vi "v4.vi"() -> ()   [LabVIEW 2015]
uses:
  <vilib>/Analysis/3filter.llb/Filter Passband Type.ctl
  <vilib>/Instr/_visa.llb/VISA Configure Serial Port (Instr).vi
  <vilib>/Analysis/3filter.llb/Butterworth Filter (DBL).vi
  <vilib>/Analysis/NI_AALBase.lvlib
panel:
  in  "Tab Control":enum32{"Configurações", "Gráficos"}(tab)
  in  "stop":bool
  in  "PORTA COM":refnum<visa-resource-name>
  in  "Digite aqui o endereço e nome do arquivo":string
  out "Max_Direito":dbl format="%#_3g"
  out "Max_esquerdo":dbl format="%#_3g"
  out "Angulo_E":dbl format="%#_3g"
  out "Tempo_D":dbl format="%#_3g"
  out "Angulo_D":dbl format="%#_3g"
  out "Tempo_E":dbl format="%#_3g"
  in  "milliseconds to wait":u32=1000
  out "Left":cluster{"X":dbl[], "Y":dbl[]}[](graph)
  out "Right":cluster{"X":dbl[], "Y":dbl[]}[](graph)
  out "angle 2":cluster{"X":dbl[], "Y":dbl[]}[](graph)
  out "angle_fil":dbl[](array[numeric])
  out "right_fil":dbl[](array[numeric])
  out "angle":dbl[](array[numeric])
  out "right":dbl[](array[numeric])
  out "left_Fil":dbl[](array[numeric])
  out "left":dbl[](array[numeric])
  out "Tempo":dbl[](array[numeric])
  out "Array_left":dbl[](array[numeric])
  out "Array_right":dbl[](array[numeric])
  out "Array_angle":dbl[](array[numeric])
  out "Tempo1":dbl[](array[numeric])
  # "Tempo para começar (ms)"
  # "Direito"
  # "Esquerdo"
  # "FORÇA MÁX."
  # "ÂNGULO"
  # "TEMPO"
  # "Desenvolvido por Tércio Apolinário-Souza"
  # "Esquerdo"
  # "Direito"
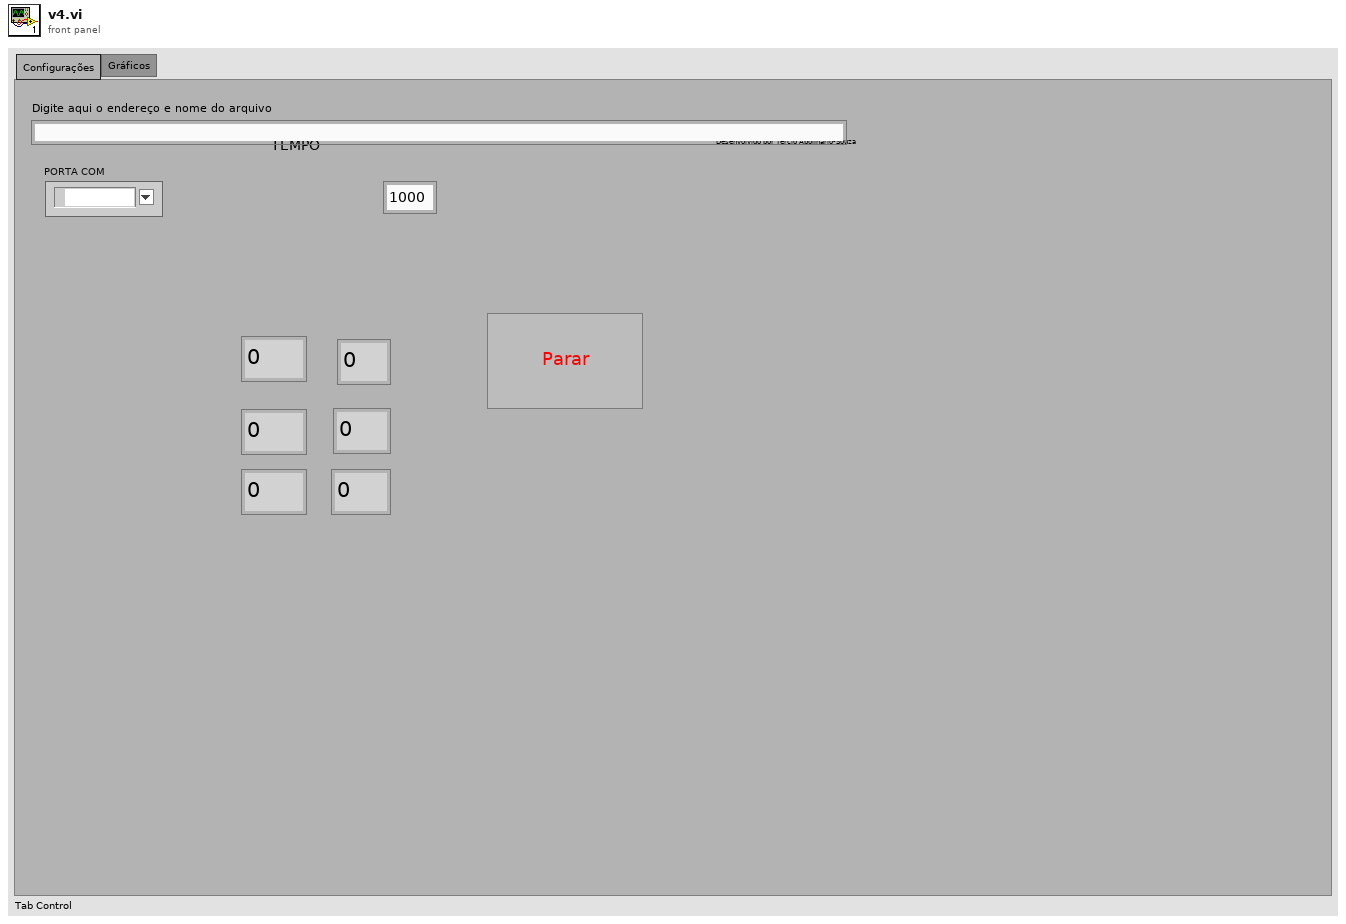
[diagram p1: front panel]
types:
  T1 = typedef "NI_AALBase.lvlib/Filter Passband Type.ctl" = enum32{"Lowpass", "Highpass", "Bandpass", "Bandstop"}
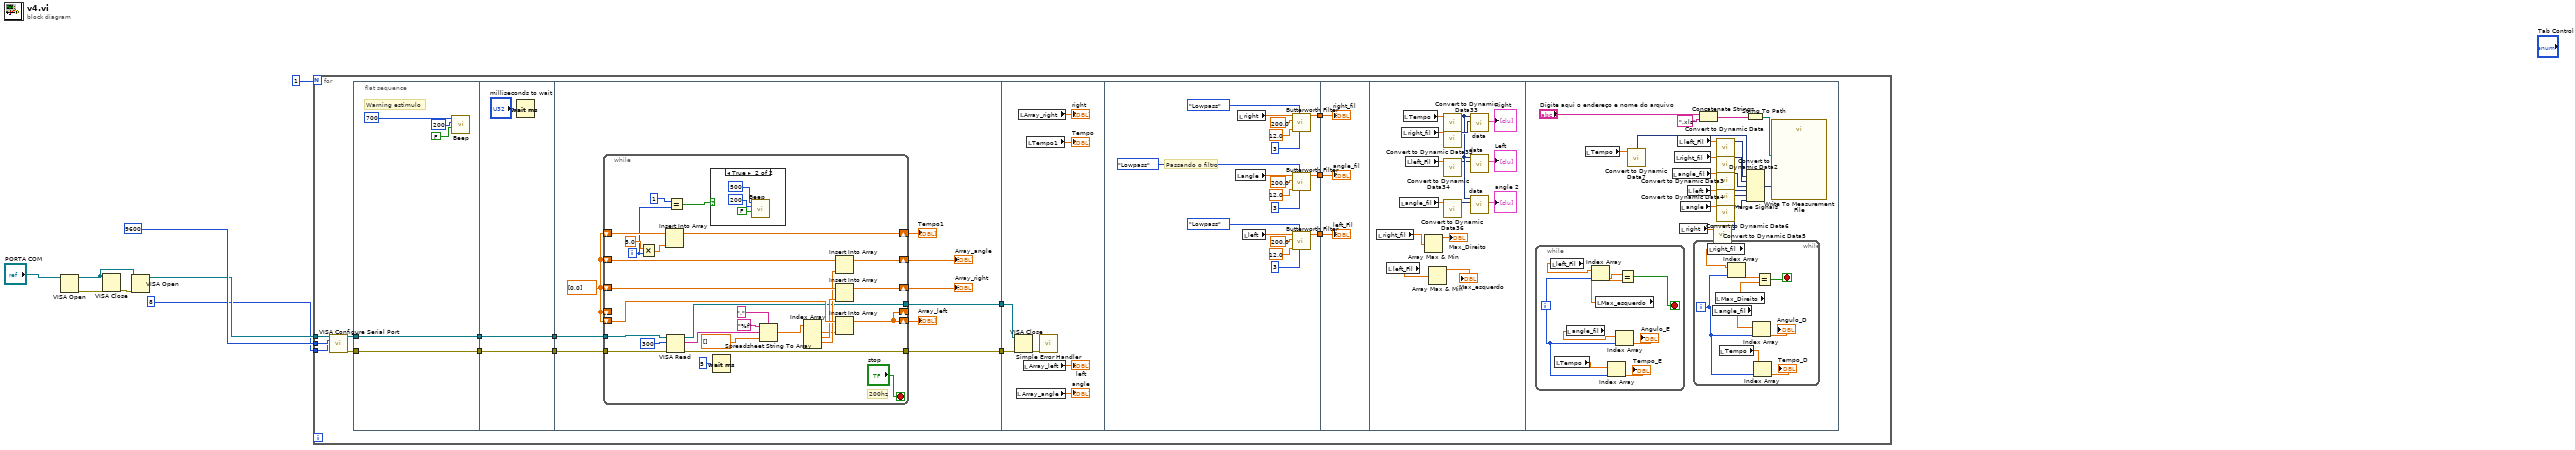
[diagram p0: block diagram]
diagram:
  n1 = VISA Open(VISA resource name="PORTA COM") -> (VISA resource name=w6:refnum<visa-resource-name>, error out=w5:errorcluster)  [unwired: 4 in]
  n2 = VISA Close(VISA resource name=w6, error in (no error)=w5) -> (error out=w4:errorcluster)
  n3 = VISA Open(error in (no error)=w4, VISA resource name=w6) -> (VISA resource name=w3:refnum<visa-resource-name>)  [unwired: 3 in, 1 out]
  n4 = for {
    N: 1 -> [_]
    tunnel: u32 9600 ("baud rate (9600)") -> [w22]
    tunnel: w3 -> [w21]
    tunnel: u16 8 ("data bits (8)") -> [w20]
    n5 = call-poly "VISA Configure Serial Port"("VISA resource name"=w21, "baud rate (9600)"=w22, "data bits (8)"=w20) -> ("VISA resource name out"=w19:refnum<visa-resource-name>, "error out"=w18:errorcluster)  [unwired: 11 in]
    n6 = flat-sequence {
      tunnel: [w23] -> w12
      tunnel: [w24] -> w11
      tunnel: w19 -> [w24]
      tunnel: w18 -> [w23]
      tunnel: w12 -> [w30]
      tunnel: [w30] -> w10
      tunnel: w11 -> [w29]
      tunnel: [w29] -> w9
      tunnel: w9 -> [w39]
      tunnel: [w37] -> w17
      tunnel: w10 -> [w38]
      tunnel: [w36] -> w16
      tunnel: w17 -> [w76]
      tunnel: w16 -> [w75]
      tunnel: [w80] -> w15
      tunnel: [w79] -> w14
      tunnel: [w78] -> w13
      tunnel: w15 -> [w98]
      tunnel: w14 -> [w97]
      tunnel: w13 -> [w96]
      frame #0 {
        # "Warning estimulo"
        n7 = call <vilib>:"Beep.vi"("use system alert? (T)"=FALSE, "duration (msec)"=u32 200, "frequency (Hz)"=u32 700) -> ()  [unwired: 9 in]
      }
      frame #1 {
        n8 = Wait (ms)(milliseconds to wait="milliseconds to wait") -> ()  [unwired: 1 out]
      }
      frame #2 {
        w32 = dbl[] [0.0] ("appended array")
        n9 = while {
          tunnel: w39 -> [w64]
          tunnel: w38 -> [w63]
          tunnel: [w50] -> w37
          tunnel: [w62] -> w36
          shift-right: [w46] -> w33
          shift-left: w32 -> [w59]
          shift-right: [w51] -> w34
          shift-left: w32 -> [w57]
          shift-right: [w49] -> w35
          shift-left: w32 -> [w56]
          shift-right: [w52] -> w31
          shift-left: w32 -> [w48]
          shift-right: [w46] -> _
          shift-left: w32 -> [_]
          i -> [w42]
          stop <- "stop" stop-if-true
          # "200hz"
          n10 = Multiply(x=5.0, y=w42) -> (x*y=w45:dbl)
          n11 = Insert Into Array(array=w48, new element=w45) -> (w52:dbl[])  [unwired: 1 in]
          n12 = VISA Read(VISA resource name=w64, byte count=u32 300, error in (no error)=w63) -> (VISA resource name out=w50:refnum<visa-resource-name>, read buffer=w60:string, error out=w62:errorcluster)  [unwired: 1 out]
          n13 = Equal?(x=1, y=w42) -> (x = y?=w40:bool)
          n14 = case shown="True" w40 {
            frame False {
            }
            frame True {
              n15 = call <vilib>:"Beep.vi"("use system alert? (T)"=FALSE, "duration (msec)"=u32 200, "frequency (Hz)"=u32 500) -> ()  [unwired: 9 in]
            }
          }
          n16 = Wait (ms)(milliseconds to wait=u32 5 ("millisecond multiple")) -> ()  [unwired: 1 out]
          n17 = Spreadsheet String To Array(delimiter (Tab)=",", format string="%f", spreadsheet string=w60, array type (2D Dbl)=dbl[] []) -> (array=w54:dbl[])
          n18 = Index Array(array=w54) -> (element #1=w53:dbl, element #2=w58:dbl, element #3=w55:dbl)  [unwired: 4 in, 1 out]
          n19 = Insert Into Array(array=w56, new element=w55) -> (w49:dbl[])  [unwired: 1 in]
          n20 = Insert Into Array(array=w57, new element=w58) -> (w51:dbl[])  [unwired: 1 in]
          n21 = Insert Into Array(array=w59, new element=w53) -> (w46:dbl[])  [unwired: 1 in]
        }
        "Tempo1" <- w31
        "Array_angle" <- w35
        "Array_right" <- w34
        "Array_left" <- w33
      }
      frame #3 {
        n22 = VISA Close(VISA resource name=w76, error in (no error)=w75) -> (error out=w77:errorcluster)
        n23 = local read "Array_angle"() -> (→"angle":dbl[])
        n24 = local read "Array_right"() -> (→"right":dbl[])
        n25 = local read "Array_left"() -> (→"left":dbl[])
        n26 = local read "Tempo1"() -> (→"Tempo":dbl[])
        n27 = call <vilib>:"Simple Error Handler.vi"("error in (no error)"=w77) -> ()  [unwired: 1 in, 8 out]
      }
      frame #4 {
        # "Passando o filtro"
        n28 = local read "angle"() -> (w81:dbl[])
        n29 = local read "right"() -> (w82:dbl[])
        n30 = local read "left"() -> (w91:dbl[])
        n31 = call-poly <vilib>:"Butterworth Filter.vi"("order"=3, "filter type"=Filter_Passband_Type."Lowpass", "low cutoff freq: fl"=12.0, "sampling freq: fs"=200.0, "X"=w82) -> ("Filtered X"=w79:dbl[])  [unwired: 3 in, 1 out]
        n32 = call-poly <vilib>:"Butterworth Filter.vi"("order"=3, "filter type"=Filter_Passband_Type."Lowpass", "low cutoff freq: fl"=12.0, "sampling freq: fs"=200.0, "X"=w81) -> ("Filtered X"=w78:dbl[])  [unwired: 3 in, 1 out]
        n33 = call-poly <vilib>:"Butterworth Filter.vi"("order"=3, "filter type"=Filter_Passband_Type."Lowpass", "low cutoff freq: fl"=12.0, "sampling freq: fs"=200.0, "X"=w91) -> ("Filtered X"=w80:dbl[])  [unwired: 3 in, 1 out]
      }
      frame #5 {
        "left_Fil" <- w98
        "right_fil" <- w97
        "angle_fil" <- w96
      }
      frame #6 {
        n34 = local read "right_fil"() -> (w102:dbl[])
        n35 = local read "left_Fil"() -> (w100:dbl[])
        n36 = local read "angle_fil"() -> (w103:dbl[])
        n37 = local read "right_fil"() -> (w104:dbl[])
        n38 = local read "Tempo"() -> (w106:dbl[])
        n39 = local read "left_Fil"() -> (w105:dbl[])
        n40 = Array Max & Min(array=w102) -> (max value=→"Max_Direito":dbl)  [unwired: 3 out]
        n41 = Array Max & Min(array=w100) -> (max value=→"Max_esquerdo":dbl)  [unwired: 3 out]
        n42 = call "Convert to Dynamic Data33"("Array"=w106) -> ("Dynamic Data Type"=w111:dynamicdata)  [unwired: 3 in]
        n43 = call "Convert to Dynamic Data35"("Array"=w104) -> ("Dynamic Data Type"=w113:dynamicdata)  [unwired: 3 in]
        n44 = call "Convert to Dynamic Data34"("Array"=w105) -> ("Dynamic Data Type"=w107:dynamicdata)  [unwired: 3 in]
        n45 = call "Convert to Dynamic Data36"("Array"=w103) -> ("Dynamic Data Type"=w112:dynamicdata)  [unwired: 3 in]
        n46 = call "data"("Y Input"=w113, "X Input"=w111) -> ("XY Graph"=→"Right":cluster{"X":dbl[], "Y":dbl[]}[])  [unwired: 8 in, 1 out]
        n47 = call "data"("Y Input"=w107, "X Input"=w111) -> ("XY Graph"=→"Left":cluster{"X":dbl[], "Y":dbl[]}[])  [unwired: 8 in, 1 out]
        n48 = call "data"("Y Input"=w112, "X Input"=w111) -> ("XY Graph"=→"angle 2":cluster{"X":dbl[], "Y":dbl[]}[])  [unwired: 8 in, 1 out]
      }
      frame #7 {
        n49 = while {
          i -> [w143]
          stop <- w147 stop-if-true
          n50 = local read "left_Fil"() -> (w150:dbl[])
          n51 = local read "Tempo"() -> (w144:dbl[])
          n52 = local read "angle_fil"() -> (w146:dbl[])
          n53 = Index Array(array=w150, index=w143) -> (element=w149:dbl)
          n54 = local read "Max_esquerdo"() -> (w148:dbl)
          n55 = Index Array(array=w144, index=w143) -> (element=→"Tempo_E":dbl)
          n56 = Index Array(array=w146, index=w143) -> (element=→"Angulo_E":dbl)
          n57 = Equal?(x=w149, y=w148) -> (x = y?=w147:bool)
        }
        n58 = local read "Tempo"() -> (w115:dbl[])
        n59 = call "Convert to Dynamic Data7"("Array"=w115) -> ("Dynamic Data Type"=w114:dynamicdata)  [unwired: 3 in]
        n60 = local read "angle_fil"() -> (w123:dbl[])
        n61 = local read "right_fil"() -> (w125:dbl[])
        n62 = local read "left_Fil"() -> (w127:dbl[])
        n63 = local read "right"() -> (w119:dbl[])
        n64 = local read "angle"() -> (w117:dbl[])
        n65 = local read "left"() -> (w121:dbl[])
        n66 = while {
          i -> [w134]
          stop <- w138 stop-if-true
          n67 = local read "right_fil"() -> (w141:dbl[])
          n68 = local read "angle_fil"() -> (w137:dbl[])
          n69 = local read "Max_Direito"() -> (w139:dbl)
          n70 = local read "Tempo"() -> (w135:dbl[])
          n71 = Index Array(array=w141, index=w134) -> (element=w140:dbl)
          n72 = Index Array(array=w137, index=w134) -> (element=→"Angulo_D":dbl)
          n73 = Index Array(array=w135, index=w134) -> (element=→"Tempo_D":dbl)
          n74 = Equal?(x=w140, y=w139) -> (x = y?=w138:bool)
        }
        n75 = Concatenate Strings("Digite aqui o endereço e nome do arquivo", ".xls" ("string")) -> (w129:string)
        n76 = call "Convert to Dynamic Data5"("Array"=w119) -> ("Dynamic Data Type"=w118:dynamicdata)  [unwired: 3 in]
        n77 = call "Convert to Dynamic Data"("Array"=w127) -> ("Dynamic Data Type"=w126:dynamicdata)  [unwired: 3 in]
        n78 = call "Convert to Dynamic Data2"("Array"=w125) -> ("Dynamic Data Type"=w124:dynamicdata)  [unwired: 3 in]
        n79 = call "Convert to Dynamic Data3"("Array"=w123) -> ("Dynamic Data Type"=w122:dynamicdata)  [unwired: 3 in]
        n80 = call "Convert to Dynamic Data4"("Array"=w121) -> ("Dynamic Data Type"=w120:dynamicdata)  [unwired: 3 in]
        n81 = call "Convert to Dynamic Data6"("Array"=w117) -> ("Dynamic Data Type"=w116:dynamicdata)  [unwired: 3 in]
        n82 = String To Path(string=w129) -> (path=w128:path)
        n83 = Merge Signals(w114, w126, w124, w122, w120, w118, w116) -> (w132:dynamicdata)
        n84 = call "Write To Measurement File"("Signals"=w132, "Filename"=w128) -> ()  [unwired: 15 in, 3 out]
      }
    }
  }
